vi "Get Plugins Status.vi"(8 "error in (no error)":errorcluster, 11 "CIF_UI in":refnum<class "CIF_UI.lvclass">) -> (0 "error out":errorcluster, 1 "Plugin Summary Info":T4[](array[typedef]), 2 "Channels":T1[][](array[typedef]), 3 "CIF_UI out":refnum<class "CIF_UI.lvclass">)   [LabVIEW 2021, in "CIF_UI.lvclass"]
uses:
  CIF_UI.lvclass
  Typedef/Plugin Summary.ctl
  Typedef/Version.ctl
  CIFCore/Grpc/CIFCoreChannel_client/RPC Messages/cif_channelcore_Channel.ctl
  CIFCore/Grpc/CIFCoreChannel_client/RPC Messages/cif_channelcore_Direction.ctl
  CIFCore/Grpc/CIFCoreChannel_client/RPC Messages/cif_channelcore_PATTERN.ctl
  CIF_UI.lvclass/CIF_UI.ctl
  <vilib>/Utility/miscctls.llb/LVMapReplaceAction.ctl
  3cb97bbe-ec67-4187-806b-96be001ee38f.vi
  <vilib>/Comparison/Less/Less Functor/Less Functor.lvclass
  CIFCore/Grpc/CIFCoreWrapper/CIFCoreWrapper.lvlib
  <vilib>/gRPC/LabVIEW gRPC Library/grpc-lvsupport-release.lvlib
  CIFCore/Grpc/CIFCoreChannel_client/CIFCoreChannel_client.lvlib
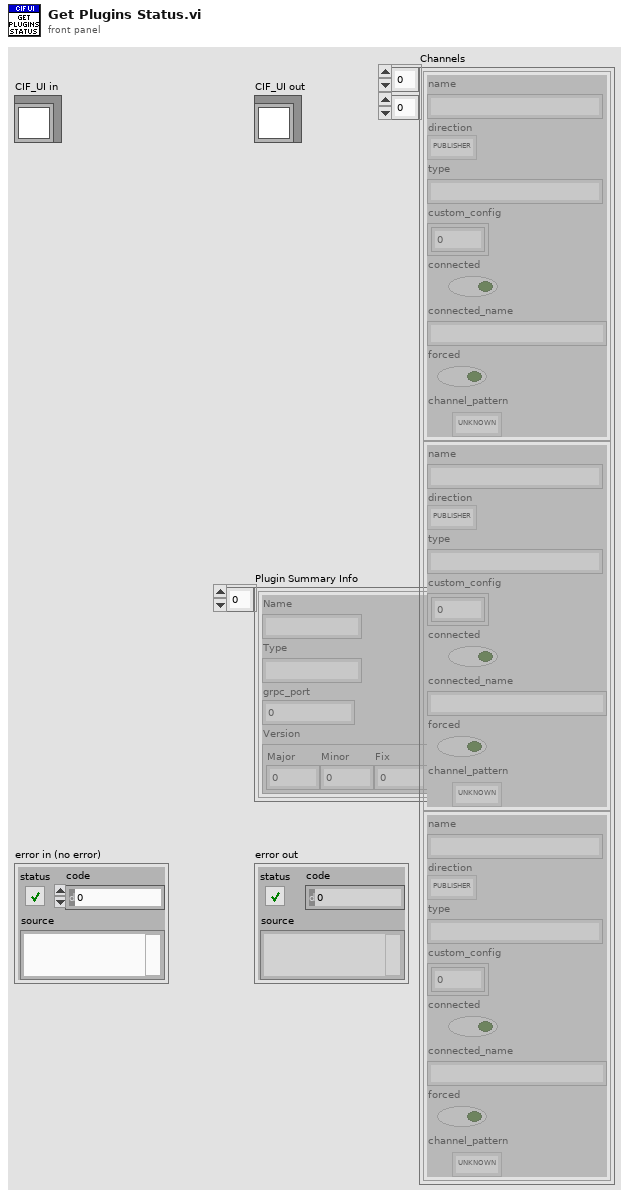
[diagram p1: front panel]
types:
  T1 = typedef "CIFCoreChannel_client.lvlib/cif_channelcore_Channel.ctl" = cluster{"name":string, "direction":T2, "type":string, "custom_config":u8[], "connected":bool, "connected_name":string, "forced":bool, "channel_pattern":T3}
  T2 = typedef "CIFCoreChannel_client.lvlib/cif_channelcore_Direction.ctl" = enum32{"PUBLISHER", "SUBSCRIBER"}
  T3 = typedef "CIFCoreChannel_client.lvlib/cif_channelcore_PATTERN.ctl" = enum32{"UNKNOWN", "TAG", "FIFO", "MULTIFIFO", "BACKPRESSUREFIFO"}
  T4 = typedef "CIF_UI.lvclass/Plugin Summary.ctl" = cluster{"Name":string, "Type":string, "grpc_port":i32, "Version":T5}
  T5 = typedef "CIF_UI.lvclass/Version.ctl" = cluster{"Major":i32, "Minor":i32, "Fix":i32}
  T6 = typedef "CIF_UI.lvclass/Plugin Connection Map.ctl" = map{string, T7}
  T7 = typedef "CIF_UI.lvclass/Plugin Connections.ctl" = cluster{"gRPC ID":T8, "Plugin Info":T9}
  T8 = typedef "grpc-lvsupport-release.lvlib/grpcId.ctl" = u64
  T9 = typedef "CIF_UI.lvclass/PluginInfo.ctl" = cluster{"Name":string, "Type":string, "grpc_port":i32, "Version":T5, "Node Status":T10}
  T10 = typedef "CIFCoreCommon.lvlib/gRPC Reported Plugin Status.ctl" = cluster{"State":T11, "Timing Statistics (us)":T12, "FIFO Statistics (us)":T14, "error":T15, "Monitor Doubles":T16, "Monitor U64":T17, "Monitor I64":T18}
  T11 = typedef "CIFCoreCommon.lvlib/Plugin State.ctl" = enum32{"Null", "Creating", "Listening", "Running", "CleaningUp", "Destroying"}
  T12 = typedef "CIFCoreCommon.lvlib/Timing Statistics.ctl" = cluster{"Period":T13, "Wake Error":T13, "Execute":T13, "Housekeep":T13, "Idle":T13, "Cleanup":T13, "Custom 1 (custom units)":T13, "Custom 2 (custom units)":T13}
  T13 = typedef "CIFCoreCommon.lvlib/Timing Stats Base.ctl" = cluster{"Max":i64, "Avg":dbl, "Min":i64}
  T14 = typedef "CIFCoreCommon.lvlib/FIFO Statistics.ctl" = cluster{"From T0":T13, "From Previous Plugin":T13, "Output Error":T13}
  T15 = typedef "CIFCoreCommon.lvlib/Simple Error.ctl" = cluster{"status":bool, "code":i32}
  T16 = typedef "CIFCoreCommon.lvlib/Monitor Doubles.ctl" = cluster{"1":dbl, "2":dbl, "3":dbl, "4":dbl}
  T17 = typedef "CIFCoreCommon.lvlib/Monitor U64.ctl" = cluster{"1":u64, "2":u64, "3":u64, "4":u64}
  T18 = typedef "CIFCoreCommon.lvlib/Monitor I64.ctl" = cluster{"1":i64, "2":i64, "3":i64, "4":i64}
  T19 = typedef "LVMapReplaceAction.ctl" = enum32{"Modify Entry only if found", "Add or Modify Entry", "Delete Entry"}
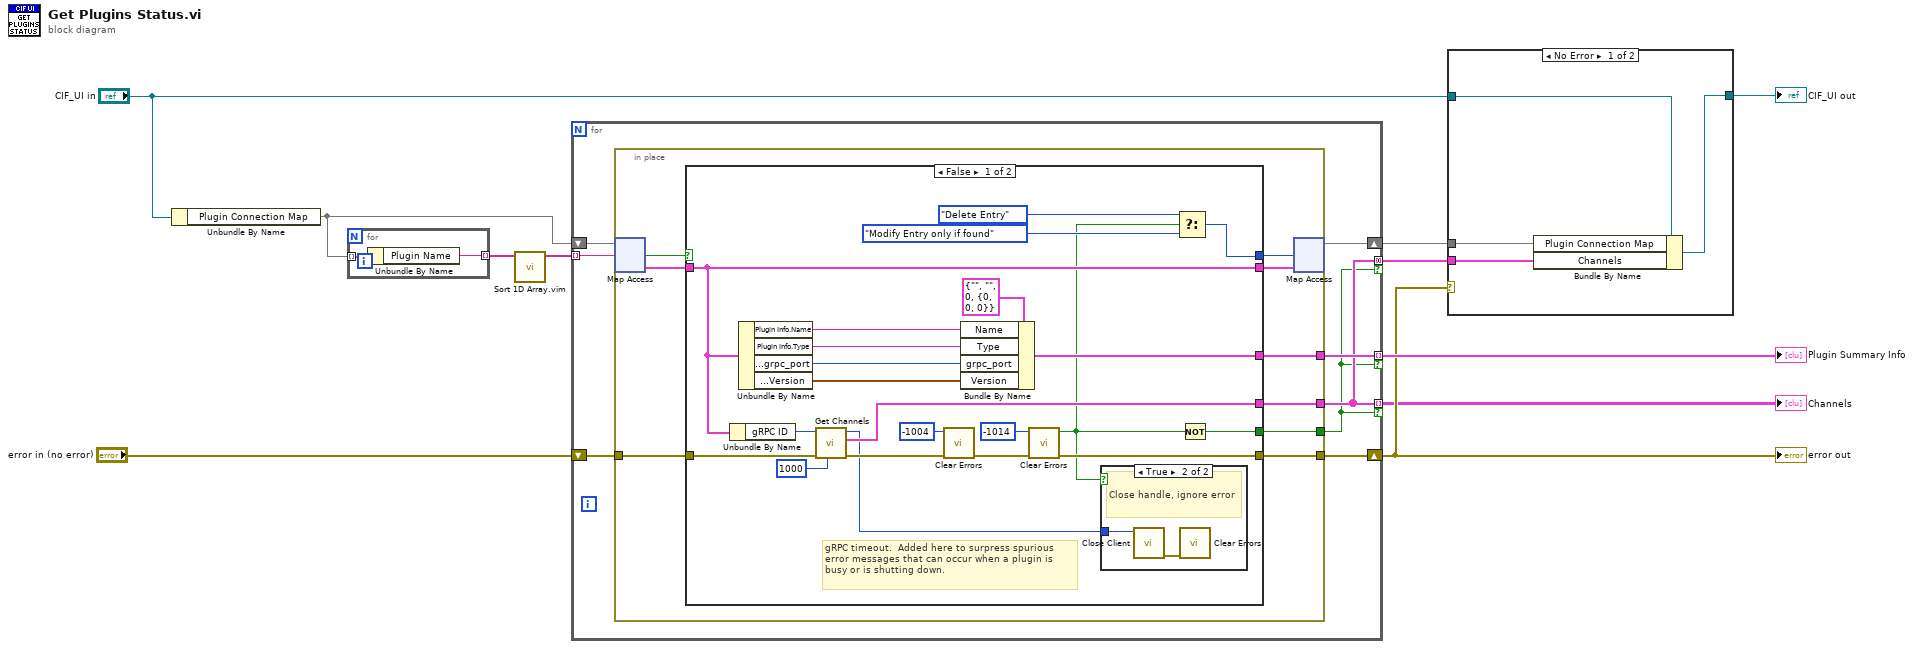
[diagram p0: block diagram]
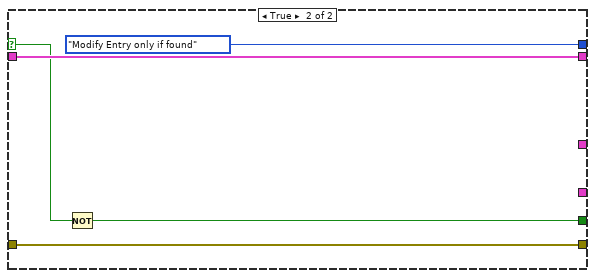
[diagram p4: hidden frame]
diagram:
  n1 = Unbundle By Name("CIF_UI in") -> ("Plugin Connection Map"=w7:T6)
  n2 = for {
    tunnel: w7 -> [w13] mode=indexing
    tunnel: [w12] -> w9 mode=indexing
    n3 = Unbundle By Name(w13) -> ("Plugin Name"=w12:string)
  }
  n4 = call "Sort 1D Array.vim"("unsorted array"=w9) -> ("sorted array"=w8:string[])  [unwired: 10 in]
  n5 = for {
    tunnel: [w20] -> w11 mode=indexing if=w14
    tunnel: [w15] -> w2 mode=indexing if=w14
    shift-right: [w21] -> w3
    shift-left: "error in (no error)" -> [w19]
    tunnel: w8 -> [w18] mode=indexing
    shift-right: [w16] -> w5
    shift-left: w7 -> [w17]
    tunnel: [w15] -> w1 mode=concatenating if=w14
    n6 = in-place {
      in-place-border: [w30] -> w21
      in-place-border: [w29] -> w20
      in-place-border: w19 -> [w28]
      in-place-border: [w27] -> w15
      in-place-border: [w22] -> w14
      n7 = in-place-map #1(w17, w18) -> (w25:T7, w26:bool)  [unwired: 1 in]
      n8 = case shown="False" w26 {
        selector: w26 -> [_ w57]
        tunnel: [w43 w56] -> w30
        tunnel: [w52 _] -> w29
        tunnel: w28 -> [w51 w56]
        tunnel: [w50 _] -> w27
        tunnel: w25 -> [w41 w59]
        tunnel: [w37 LVMapReplaceAction."Modify Entry only if found" ("action")] -> w24
        tunnel: [w41 w59] -> w23
        tunnel: [w40 w55] -> w22
        frame False {
          # "gRPC timeout.  Added here to surpress spurious error messages that can occur when a plugin is busy or is shutting down."
          n9 = Unbundle By Name(w41) -> ("gRPC ID"=w49:T8)
          n10 = Unbundle By Name(w41) -> ("Plugin Info.Name"=w47:string, "Plugin Info.Type"=w44:string, "Plugin Info.grpc_port"=w45:i32, "Plugin Info.Version"=w46:T5)
          n11 = call "Get Channels.vi"("timeout (ms)"=1000, "error in"=w51, "gRPC ID"=w49) -> ("error out"=w34:errorcluster, "Channels"=w50:T1[], "gRPC ID out"=w32:T8)  [unwired: 6 in]
          n12 = call <vilib>:"Clear Errors.vi"("error in (no error)"=w34, "specific error code to clear (0: all)"=-1004) -> ("error out"=w33:errorcluster)  [unwired: 4 in, 1 out]
          n13 = Bundle By Name(cluster=T4 {"Name"="", "Type"="", "grpc_port"=0, "Version"={"Major"=0, "Minor"=0, "Fix"=0}} ("Plugin Summary"), "Name"=w47, "Type"=w44, "grpc_port"=w45, "Version"=w46) -> (w52:T4)
          n14 = call <vilib>:"Clear Errors.vi"("error in (no error)"=w33, "specific error code to clear (0: all)"=-1014) -> ("error out"=w43:errorcluster, "specific error cleared?"=w31:bool)  [unwired: 4 in]
          n15 = case shown="True" w31 {
            tunnel: w32 -> [_ w54]
            frame False {
            }
            frame True {
              # "Close handle, ignore error"
              n16 = call <vilib>:"Close Client.vi"("ClientID in"=w54) -> ("error out"=w53:errorcluster)  [unwired: 10 in]
              n17 = call <vilib>:"Clear Errors.vi"("error in (no error)"=w53) -> ()  [unwired: 5 in, 2 out]
            }
          }
          n18 = Select(t=LVMapReplaceAction."Delete Entry" ("action"), s=w31, f=LVMapReplaceAction."Modify Entry only if found" ("action")) -> (s? t:f=w37:T19)
          n19 = Not(x=w31) -> (.not. x?=w40:bool)
        }
        frame True {
          n20 = Not(x=w57) -> (.not. x?=w55:bool)
        }
      }
      n21 = in-place-map #1(w23, w24) -> (w16:T6)  [unwired: 2 out]
    }
  }
  "error out" <- w3
  "Plugin Summary Info" <- w11
  "Channels" <- w2
  n22 = case shown="No Error" w3 {
    tunnel: "CIF_UI in" -> [w63 w64]
    tunnel: w5 -> [w62 _]
    tunnel: [w61 w64] -> w4
    tunnel: w1 -> [w60 _]
    frame No Error {
      n23 = Bundle By Name(cluster=w63, "Plugin Connection Map"=w62, "Channels"=w60) -> (w61:refnum<class "CIF_UI.lvclass">)
    }
    frame Error {
    }
  }
  "CIF_UI out" <- w4
